vi "Configure9226.vi"(7 "Channel Number":i32, 8 "error in (no error)":errorcluster, 10 "Properties":T1[](array[typedef]), 11 "IO Ref":refnum<k21>) -> (0 "error out":errorcluster, 3 "IO Ref out":refnum<k21>)   [LabVIEW 2017, in "ScanEngine.lvlib"]
uses:
  <vilib>/addons/InsightCM/Devices/Shared/Common/ScanEngine/ScanEngine.lvlib
  <vilib>/addons/InsightCM/MessageBus/Base/controls/KeyValuePair.ctl
  <resource>/objmgr/cRIO.rc
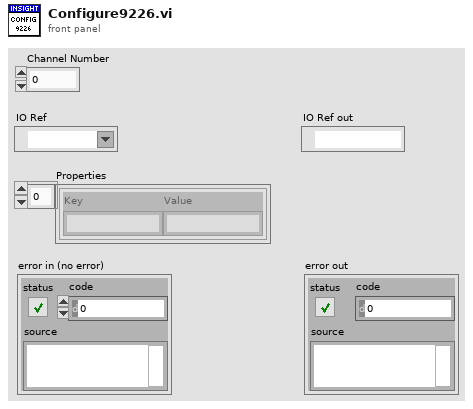
[diagram p1: front panel]
types:
  T1 = typedef "KeyValuePair.ctl" = cluster{"Key":string, "Value":string}
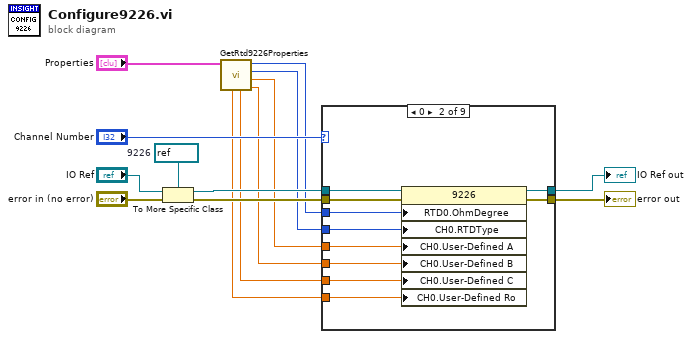
[diagram p0: block diagram]
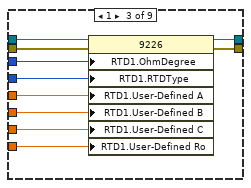
[diagram p3: hidden frame]
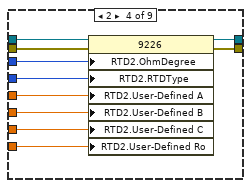
[diagram p4: hidden frame]
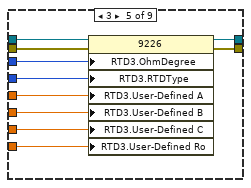
[diagram p5: hidden frame]
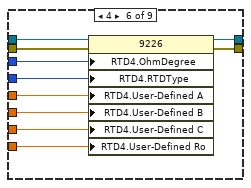
[diagram p6: hidden frame]
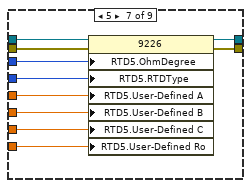
[diagram p7: hidden frame]
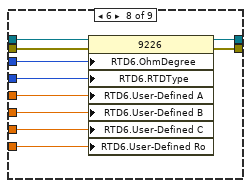
[diagram p8: hidden frame]
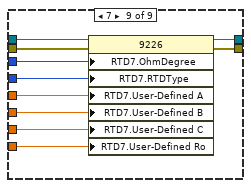
[diagram p9: hidden frame]
diagram:
  w12 = refnum<k21> refnum  # 9226
  n1 = To More Specific Class(target class=w12, reference="IO Ref", error in="error in (no error)") -> (specific class reference=w11:refnum<k21>, error out=w15:errorcluster)
  n2 = call <vilib>:"GetRtd9226Properties.vi"("Properties"="Properties") -> ("B"=w4:dbl, "A"=w5:dbl, "RTD type"=w6:u32, "RTD ohm degree range"=w7:u32, "C"=w3:dbl, "r0"=w2:dbl)  [unwired: 5 in]
  n3 = case shown="0" "Channel Number" {
    tunnel: w15 -> [w17 w24 w34 w44 w54 w64 w74 w84 w94]
    tunnel: [w17 w27 w37 w47 w57 w67 w77 w87 w97] -> w9
    tunnel: w11 -> [w16 w26 w36 w46 w56 w66 w76 w86 w96]
    tunnel: [w16 w25 w35 w45 w55 w65 w75 w85 w95] -> w14
    tunnel: w7 -> [_ w18 w33 w43 w53 w63 w73 w83 w93]
    tunnel: w6 -> [_ w19 w32 w42 w52 w62 w72 w82 w88]
    tunnel: w5 -> [_ w23 w31 w41 w51 w61 w71 w81 w92]
    tunnel: w2 -> [_ w22 w28 w38 w48 w58 w68 w78 w89]
    tunnel: w4 -> [_ w21 w30 w40 w50 w60 w70 w80 w91]
    tunnel: w3 -> [_ w20 w29 w39 w49 w59 w69 w79 w90]
    frame -1, Default {
    }
    frame 0 {
      n4 = property class="9226"(reference=w26, error in=w24, "RTD0.OhmDegree"=w18, "CH0.RTDType"=w19, "CH0.User-Defined A"=w23, "CH0.User-Defined B"=w21, "CH0.User-Defined C"=w20, "CH0.User-Defined Ro"=w22) -> (reference out=w25:refnum<k21>, error out=w27:errorcluster)
    }
    frame 1 {
      n5 = property class="9226"(reference=w36, error in=w34, "RTD1.OhmDegree"=w33, "RTD1.RTDType"=w32, "RTD1.User-Defined A"=w31, "RTD1.User-Defined B"=w30, "RTD1.User-Defined C"=w29, "RTD1.User-Defined Ro"=w28) -> (reference out=w35:refnum<k21>, error out=w37:errorcluster)
    }
    frame 2 {
      n6 = property class="9226"(reference=w46, error in=w44, "RTD2.OhmDegree"=w43, "RTD2.RTDType"=w42, "RTD2.User-Defined A"=w41, "RTD2.User-Defined B"=w40, "RTD2.User-Defined C"=w39, "RTD2.User-Defined Ro"=w38) -> (reference out=w45:refnum<k21>, error out=w47:errorcluster)
    }
    frame 3 {
      n7 = property class="9226"(reference=w56, error in=w54, "RTD3.OhmDegree"=w53, "RTD3.RTDType"=w52, "RTD3.User-Defined A"=w51, "RTD3.User-Defined B"=w50, "RTD3.User-Defined C"=w49, "RTD3.User-Defined Ro"=w48) -> (reference out=w55:refnum<k21>, error out=w57:errorcluster)
    }
    frame 4 {
      n8 = property class="9226"(reference=w66, error in=w64, "RTD4.OhmDegree"=w63, "RTD4.RTDType"=w62, "RTD4.User-Defined A"=w61, "RTD4.User-Defined B"=w60, "RTD4.User-Defined C"=w59, "RTD4.User-Defined Ro"=w58) -> (reference out=w65:refnum<k21>, error out=w67:errorcluster)
    }
    frame 5 {
      n9 = property class="9226"(reference=w76, error in=w74, "RTD5.OhmDegree"=w73, "RTD5.RTDType"=w72, "RTD5.User-Defined A"=w71, "RTD5.User-Defined B"=w70, "RTD5.User-Defined C"=w69, "RTD5.User-Defined Ro"=w68) -> (reference out=w75:refnum<k21>, error out=w77:errorcluster)
    }
    frame 6 {
      n10 = property class="9226"(reference=w86, error in=w84, "RTD6.OhmDegree"=w83, "RTD6.RTDType"=w82, "RTD6.User-Defined A"=w81, "RTD6.User-Defined B"=w80, "RTD6.User-Defined C"=w79, "RTD6.User-Defined Ro"=w78) -> (reference out=w85:refnum<k21>, error out=w87:errorcluster)
    }
    frame 7 {
      n11 = property class="9226"(reference=w96, error in=w94, "RTD7.OhmDegree"=w93, "RTD7.RTDType"=w88, "RTD7.User-Defined A"=w92, "RTD7.User-Defined B"=w91, "RTD7.User-Defined C"=w90, "RTD7.User-Defined Ro"=w89) -> (reference out=w95:refnum<k21>, error out=w97:errorcluster)
    }
  }
  "IO Ref out" <- w14
  "error out" <- w9
